vi "unflattenFromString.vi"(8 "error in (no error)":errorcluster, 10 "binary string":string, 11 "iMessage in":refnum<class "iMessage.lvclass">) -> (0 "error out":errorcluster, 3 "iMessage out":refnum<class "iMessage.lvclass">)   [LabVIEW 2017, in "Message Interface.lvlib" / "iMessage.lvclass"]
uses:
  iMessage.lvclass
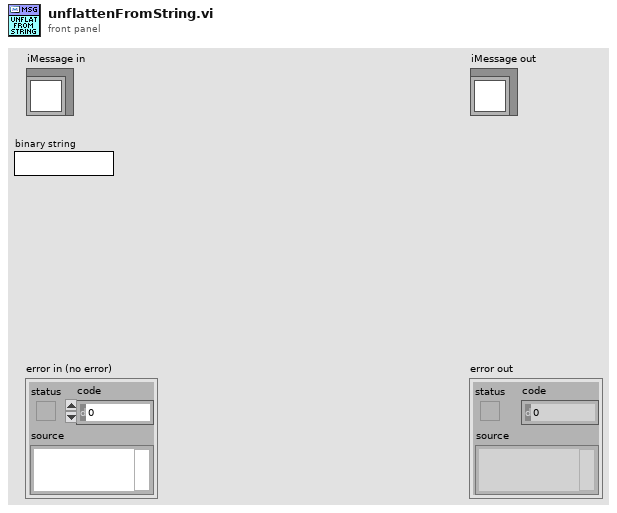
[diagram p1: front panel]
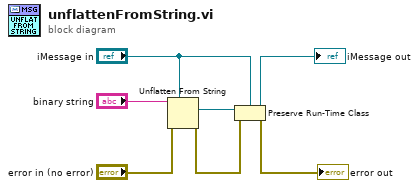
[diagram p0: block diagram]
diagram:
  n1 = Unflatten From String(type="iMessage in", binary string="binary string", error in (no error)="error in (no error)") -> (value=w3:refnum<class "iMessage.lvclass">, error out=w5:errorcluster)  [unwired: 2 in, 1 out]
  n2 = Preserve Run-Time Class(object in=w3, error in=w5, 2:"iMessage in") -> (object out=→"iMessage out":refnum<class "iMessage.lvclass">, error out=→"error out":errorcluster)
